vi "KalmanFilter.vi"() -> ()   [LabVIEW 2020]
uses:
  <vilib>/Analysis/Matrix/Datatypes/RealMatrix.ctl
  <vilib>/Analysis/Matrix/NI_Matrix.lvlib
panel:
  in  "Observations1\nGyro":dbl format="%#_13g"
  in  "Observations2\naccelerometer angle":dbl format="%#_13g"
  out "State Predicted Estimate X^(k+1/k)":dbl[](array[numeric])
  in  "Steady State Kalman Predictor Gain matrixx":T1
  in  "F  Matrix":T1
  in  "H Matrix":T1
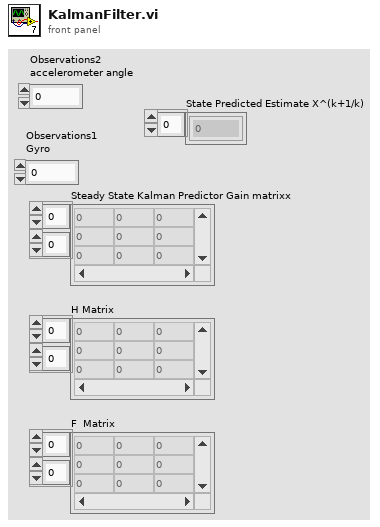
[diagram p1: front panel]
types:
  T1 = typedef "NI_Matrix.lvlib/RealMatrix.ctl" = dbl[][]
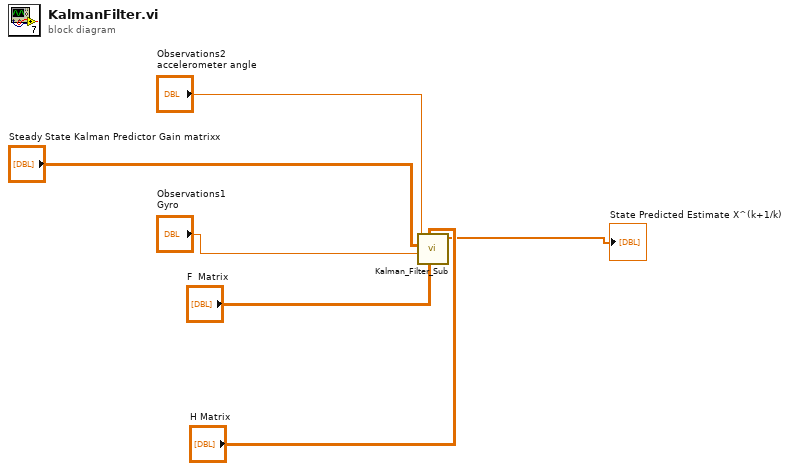
[diagram p0: block diagram]
diagram:
  n1 = call "Kalman_Filter_Sub.vi"("F  Matrix"="F  Matrix", "H Matrix"="H Matrix", "Gyro"="Observations1\nGyro", "Steady State Kalman Predictor Gain matrix"="Steady State Kalman Predictor Gain matrixx", "accelerometer angle"="Observations2\naccelerometer angle") -> ("State Predicted Estimate X^(k+1/k)"=→"State Predicted Estimate X^(k+1/k)":dbl[])  [unwired: 6 in]
